vi "Get MCS wrapper.vi"(8 "error in (no error)":errorcluster caption="错误输入（无错误）", 9 "pACKInfo":T1, 10 "dwCanNodeId":u32, 11 "dwDevIndex":u32) -> (0 "error out":errorcluster caption="错误输出", 1 "MCS":i32, 3 "function return":u32)   [LabVIEW 2016, in "UISimCanFunc_wrapper.lvlib"]
doc: "_declspec (dllexport) DWORD GetMCS_wrapper(DWORD dwDevIndex, DWORD dwCanNodeId, P_BASIC_ACK_OBJ pACKInfo);"
uses:
  <userlib>/UISimCanFunc_wrapper/UISimCanFunc_wrapper.lvlib
  <userlib>/UISimCanFunc_wrapper/UISimCanFunc_wrapper.dll
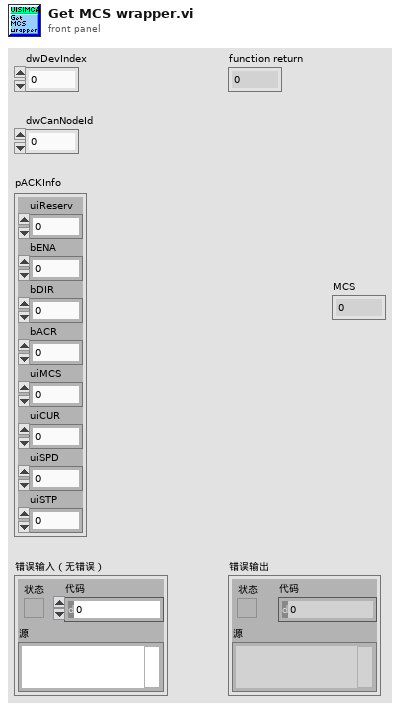
[diagram p1: front panel]
types:
  T1 = cluster{"uiReserv":u32, "bENA":i32, "bDIR":i32, "bACR":i32, "uiMCS":u32, "uiCUR":u32, "uiSPD":u32, "uiSTP":u32}
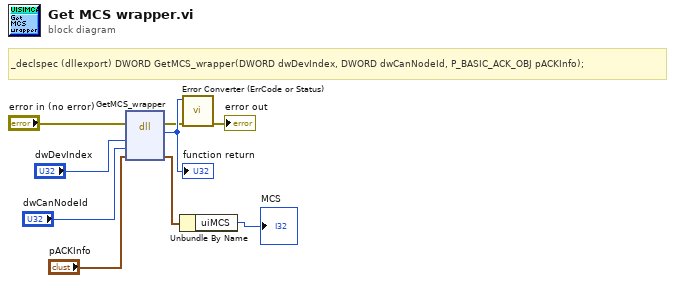
[diagram p0: block diagram]
diagram:
  # "_declspec (dllexport) DWORD GetMCS_wrapper(DWORD dwDevIndex, DWORD dwCanNodeId, P_BASIC_ACK_OBJ pACKInfo);"
  n1 = dll-call lib="C:/Program Files (x86)/National Instruments/LabVIEW 2016/user.lib/UISimCanFunc_wrapper/UISimCanFunc_wrapper.*" fn="GetMCS_wrapper"(error in="error in (no error)", "dwDevIndex"="dwDevIndex", "dwCanNodeId"="dwCanNodeId", "pACKInfo"="pACKInfo") -> (error out=w4:errorcluster, w9:u32, "pACKInfo"=w2:T1)  [unwired: 4 in, 1 out]
  "function return" <- w9
  n2 = Unbundle By Name(w2) -> ("uiMCS"=→"MCS":u32)
  n3 = call <userlib>:"Error Converter (ErrCode or Status).vi"("error in (no error)"=w4, "error code"=w9) -> ("error out"=→"error out":errorcluster)  [unwired: 9 in]
